vi "liblinear_load_model.vi"(8 "error in (no error)":errorcluster, 11 "File path":path) -> (0 "error out":errorcluster, 3 "model":T1={"liblinear_parameter"={"solver_type"=0, "eps"=0.01, "C"=1.0, "weight_label"=[], "weight"=[], "p"=0.1}, "nr_class"=0, "nr_feature"=0, "w"=[], "label"=[], "bias"=0.0} {"liblinear_parameter"."solver_type" items=["L2R_LR"=0, "L2R_L2LOSS_SVC_DUAL"=1, "L2R_L2LOSS_SVC"=2, "L2R_L1LOSS_SVC_DUAL"=3, "MCSVM_CS"=4, "L1R_L2LOSS_SVC"=5, "L1R_LR"=6, "L2R_LR_DUAL"=7, "L2R_L2LOSS_SVR"=11, "L2R_L2LOSS_SVR_DUAL"=12, "L2R_L1LOSS_SVR_DUAL"=13]})   [LabVIEW 2015]
uses:
  Controls/liblinear_model.ctl
  Controls/liblinear_parameter.ctl
  Controls/liblinear_solver.ctl
  bin/x64/LabVIEW-liblinear.dll
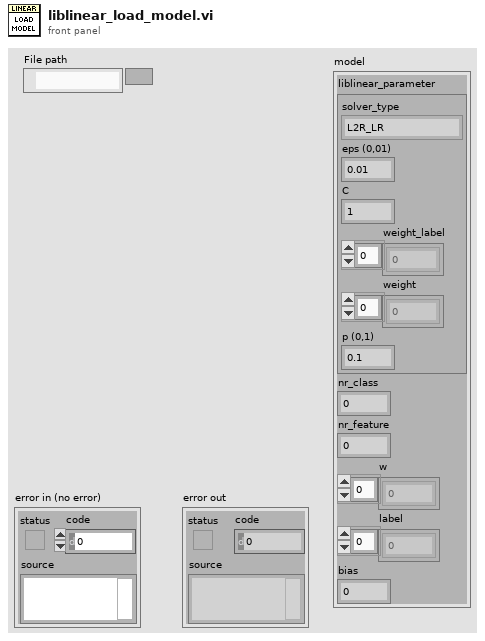
[diagram p1: front panel]
types:
  T1 = typedef "liblinear_model.ctl" = cluster{"liblinear_parameter":T2, "nr_class":i32, "nr_feature":i32, "w":dbl[], "label":i32[], "bias":dbl}
  T2 = typedef "liblinear_parameter.ctl" = cluster{"solver_type":T3, "eps":dbl, "C":dbl, "weight_label":i32[], "weight":dbl[], "p":dbl}
  T3 = typedef "liblinear_solver.ctl" = u32
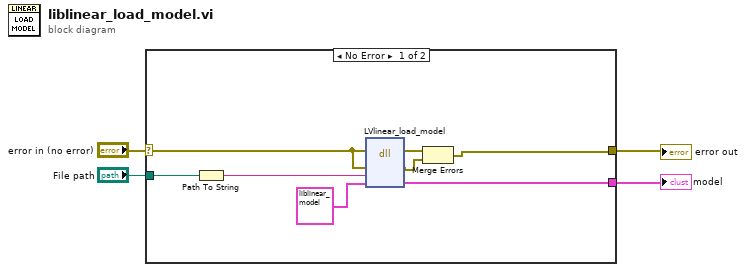
[diagram p0: block diagram]
diagram:
  n1 = case shown="No Error" "error in (no error)" {
    selector: "error in (no error)" -> [w10 w13]
    tunnel: [w9 w13] -> w4
    tunnel: "File path" -> [w12 _]
    tunnel: [w8 _] -> w1
    frame No Error {
      n2 = Path To String(path=w12) -> (string=w11:string)
      n3 = dll-call lib="C:/dev/LabVIEW-libsvm/LabVIEW/bin/x64/LabVIEW-liblinear.*" fn="LVlinear_load_model"(error in=w10, "lvErr"=w10, "path_in"=w11, "model_in"=T1 {"liblinear_parameter"={"solver_type"=0, "eps"=0.01, "C"=1.0, "weight_label"=[], "weight"=[], "p"=0.1}, "nr_class"=0, "nr_feature"=0, "w"=[], "label"=[], "bias"=0.0} ("model")) -> (error out=w7:errorcluster, "lvErr"=w6:errorcluster, "model_in"=w8:T1)  [unwired: 4 in, 1 out]
      n4 = Merge Errors(w7, w6) -> (w9:errorcluster)
    }
    frame Error {
    }
  }
  "error out" <- w4
  "model" <- w1
